vi "write_file_test_4loop_1.vi"() -> ()   [LabVIEW 2016]
uses:
  <vilib>/Utility/file.llb/Write Delimited Spreadsheet (DBL).vi
  <vilib>/LabVIEW Interface for Arduino/LabVIEW Interface for Arduino.lvlib
panel:
  in  "y":i32=100
  out "Voltage":dbl(knob) scale=0.0..5.0
  out "Numeric":i32
  in  "transpose? (no:F) 2":bool
  in  "append to file? (new file:F) 2":bool
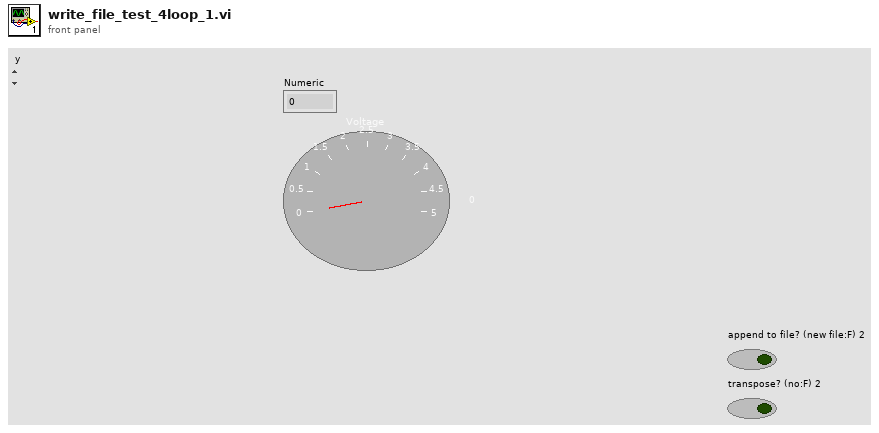
[diagram p1: front panel]
types:
  T1 = typedef "LabVIEW Interface for Arduino.lvlib/Arduino Resource.ctl" = cluster{"VISA resource":refnum<visa-resource-name>, "Board Type":T2, "Connection Type":enum8{"USB / Serial"}, "Bytes Per Packet (15)":u8}
  T2 = typedef "LabVIEW Interface for Arduino.lvlib/Board Type.ctl" = enum16{"Uno", "Dimuelanove w/Atmega 328", "Mega 2560"}
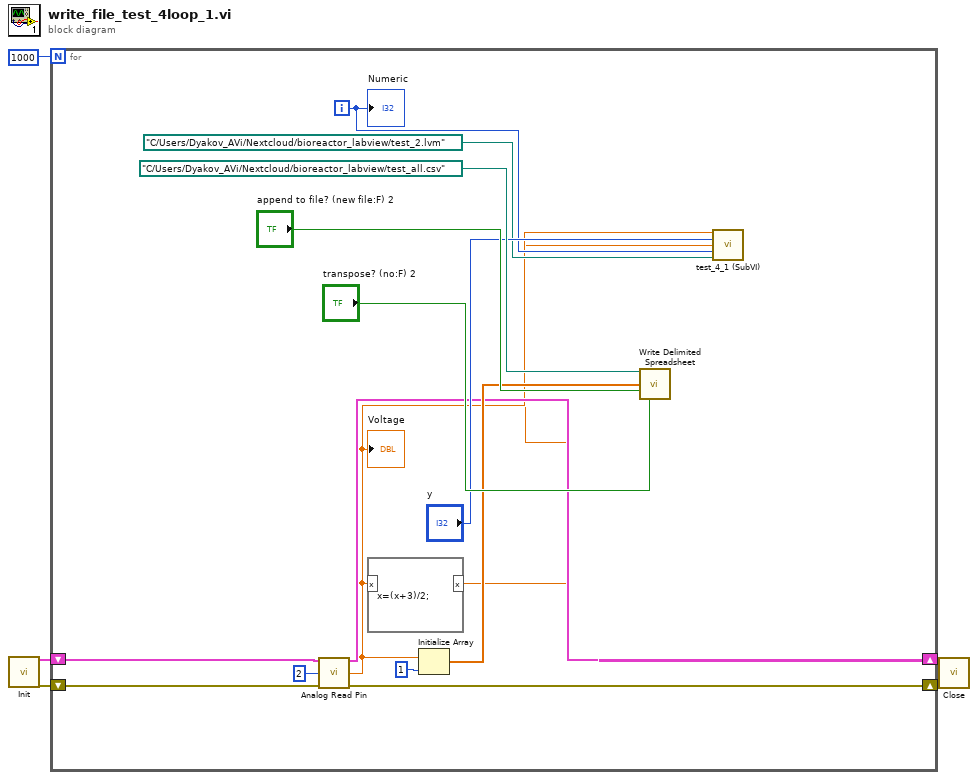
[diagram p0: block diagram]
diagram:
  n1 = call <vilib>:"Init.vi"() -> ("Arduino Resource"=w5:T1, "error out"=w4:errorcluster)  [unwired: 18 in]
  n2 = for {
    N: 1000 -> [_]
    shift-right: [w10] -> w2
    shift-left: w5 -> [w14]
    shift-right: [w9] -> w1
    shift-left: w4 -> [w13]
    i -> [w12]
    n3 = call <vilib>:"Analog Read Pin.vi"("Arduino Resource"=w14, "Analog Input Pin (0)"=u8 2, "error in"=w13) -> ("Arduino Resource"=w10:T1, "Voltage"=w7:dbl, "error out"=w9:errorcluster)  [unwired: 10 in]
    "Voltage" <- w7
    n4 = formula code="x=(x+3)/2;"("x"=w7) -> ("x"=w6:dbl)
    n5 = Initialize Array(w7, 1 ("dimension size")) -> (w11:dbl[])
    n6 = call-poly <vilib>:"Write Delimited Spreadsheet.vi"("file path (dialog if empty)"=path "C:/Users/Dyakov_AVi/Nextcloud/bioreactor_labview/test_all.csv", "1D data"=w11, "append to file? (new file:F)"="append to file? (new file:F) 2", "transpose? (no:F)"="transpose? (no:F) 2") -> ()  [unwired: 10 in, 2 out]
    n7 = call "test_4_1 (SubVI).vi"("Voltage"=w7, "y"="y", "Lux"=w6, "Numeric"=w12, "Filename"=path "C:/Users/Dyakov_AVi/Nextcloud/bioreactor_labview/test_2.lvm") -> ()  [unwired: 11 in]
    "Numeric" <- w12
  }
  n8 = call <vilib>:"Close.vi"("Arduino Resource"=w2, "error in"=w1) -> ()  [unwired: 13 in, 1 out]
